vi "运维调试_采配水V4.vi"() -> ()   [LabVIEW 2016, in "PLC.lvlib"]
uses:
  PLC.lvlib
  <vilib>/Plasmionique/MB Master/MB_Master/MB_Master.lvclass
  <vilib>/Utility/miscctls.llb/LVPointTypeDef.ctl
  <vilib>/Plasmionique/MB Master/MB_Master_Serial/MB_Master_Serial.lvclass
  C:/Program Files (x86)/National Instruments/LabVIEW 2016/vi.lib/Plasmionique/MB Master/MB_Master/MB_Master.lvclass
  <vilib>/Instr/_visa.llb/VISA Configure Serial Port (Instr).vi
  <vilib>/NI/Modbus Library/API/Wrapper/Create TCP Slave.vi
  <vilib>/NI/Modbus Library/API/slave/Modbus Slave.lvclass
  <vilib>/Plasmionique/MB Master/MB Master.lvlib
  <vilib>/ptbypt/NI_PtbyPt.lvlib
  <vilib>/NI/Modbus Library/API/Wrapper/API Main.lvlib
panel:
  out "R111":i16 caption="三级水样池润洗时间"
  in  "三级过滤系统":bool
  out "R110":i16 caption="集气时间"
  out "R104":i16 caption="三级润洗时间"
  out "R103":i16 caption="二级润洗时间"
  out "R107":i16 caption="进气时间"
  out "R43":u16
  in  "Y30":bool
  out "Registers":u16[](array[numeric])
  out "R124":i16 caption="加标回收配水时间"
  out "R42":i16
  in  "Y29":bool
  in  "更新程序":bool
  out "R122":i16 caption="二级自来水清洗时间"
  out "R121":i16 caption="一级自来水清洗时间"
  out "R120":i16 caption="过滤自来水清洗时间"
  out "清洗次数":u16
  out "当前启动泵号":u16(ring) items=["1号泵", "2号泵"]
  out "R116":i16 caption="储水时间"
  in  "R113":u16(ring) caption="水箱储水水体" items=["自来水", "水样"]
  out "R112":i16 caption="二级水样池进样超时"
  out "R31":u16
  out "R30":u16
  out "R29":u16
  out "R28":u16
  out "R27":u16
  out "R26":u16
  out "R25":u16
  out "R24":u16
  out "R23":u16
  out "R22":u16
  out "R21":u16
  out "R20":u16
  out "R19":u16
  out "R18":u16
  out "R17":u16
  out "R16":u16
  out "R15":u16
  out "R14":u16
  out "R13":u16
  out "压力传感器":dbl format="%#.2f"
  in  "Y18":bool
  in  "Y17":bool
  in  "Y14":bool
  in  "Y13":bool
  in  "Y1":bool
  in  "Y0":bool
  in  "Y12":bool
  in  "Y11":bool
  in  "Y10":bool
  in  "Y9":bool
  in  "Y8":bool
  in  "Y7":bool
  out "X2":bool caption="X1"
  out "采配水版本号":string
  out "R117":i16 caption="清洗频次设定"
  out "通讯故障":bool
  in  "R100":u16(ring) caption="采水泵工作模式" items=["泵1单泵单管路", "泵2单泵单管路", "潜水泵双泵双管路", "自吸泵双泵双管路"]
  out "X10":bool caption="氨氮水样池液位开关SL3"
  out "X9":bool caption="泵2过载报警_KM2"
  out "X8":bool caption="泵1过载报警_KM1"
  out "X7":bool caption="断电检测_PA"
  out "X6":bool caption="门禁开关_AS"
  out "X5":bool caption="烟雾检测_SA"
  out "X4":bool caption="浸水检测_WIA"
  out "X3":bool caption="水流开关_FS"
  out "X1":bool
  out "X0":bool caption="采样池液位开关_SL1"
  out "R109":i16 caption="外部反冲洗时间"
  out "集成报警信息":string
  out "R108":i16 caption="进样超时时间"
  out "R106":i16 caption="排液时间"
  out "R105":i16 caption="常规模式配水时间"
  out "R102":i16 caption="沉淀时间"
  out "R101":i16 caption="一级润洗时间"
  out "R2":i16
  out "R1":i16
  out "多列列表框":i32(listbox)
  in  "Y6":bool
  in  "Y5":bool
  in  "Y4":bool
  in  "Y3":bool
  in  "Y2":bool
  in  "Y16":bool
  in  "Y15":bool
  in  "返回":bool
  in  "参数设置":bool
  in  "单步启动":bool
  in  "启动":bool
  in  "停止":bool
  # "流程计时："
  # "s"
  # "压力传感器："
  # "MPa"
  # "二级液位开关低_SL2L"
  # "二级液位开关高_SL2H"
  # "S"
  # "S"
  # "S"
  # "S"
  # "S"
  # "S"
  # "S"
  # "S"
  # "S"
  # "S"
  # "S"
  # "次"
  # "S"
  # "S"
  # "S"
  # "S"
  # "S"
  # "S"
  # "单步计时："
  # "s"
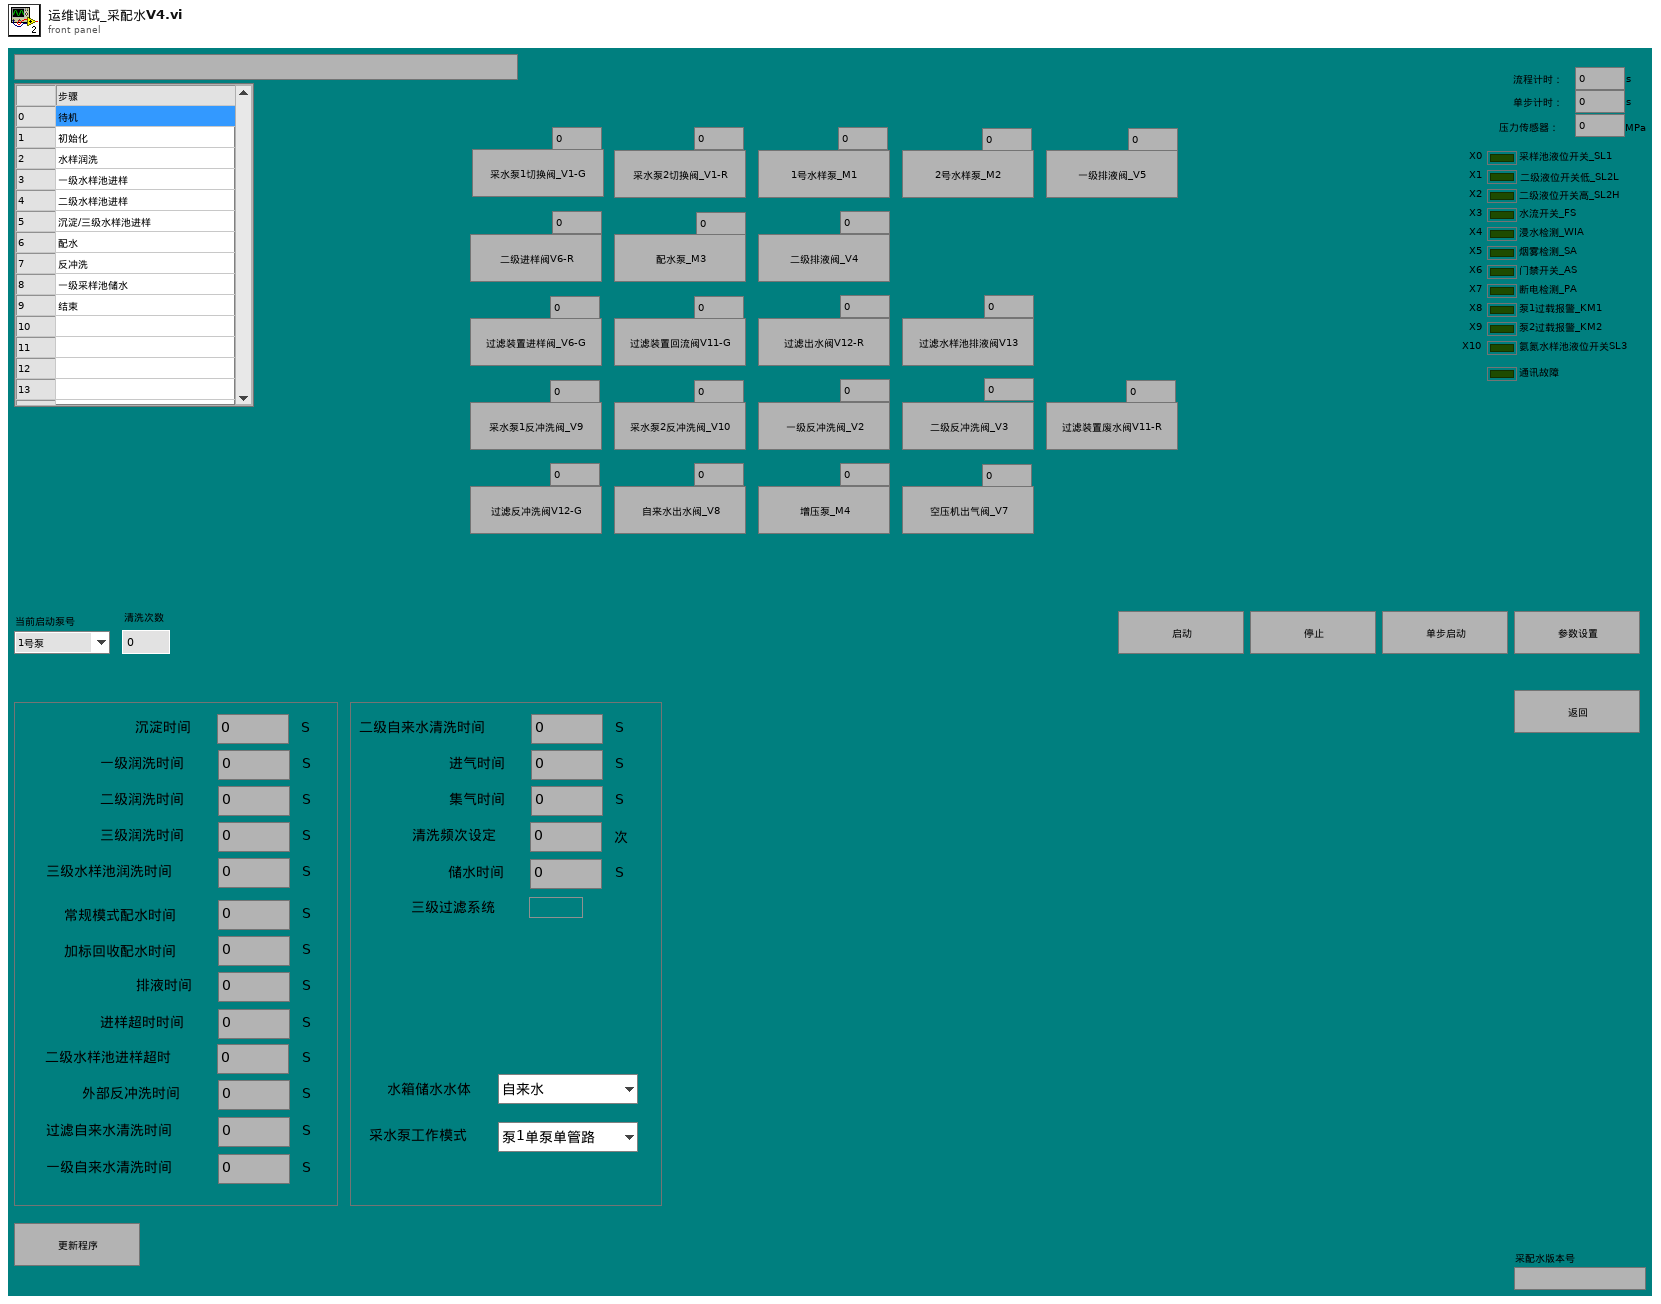
[diagram p1: front panel]
types:
  T1 = typedef "LVPointTypeDef.ctl" = cluster{"Horizontal":i16, "Vertical":i16}
  T2 = cluster{"命令":string, "数据":cluster{"starting address":u16, "holding register value":u16}}
  T3 = cluster{"时间标识":timestamp, "设备":string, "日志信息":string}
  T4 = cluster{"R0":i16, "R1":i16, "R2":i16, "R3":i16, "R4":i16, "R5":i16, "R6":i16, "R7":i16, "R8":i16, "R9":i16, "R10":i16, "R11":i16, "R12":i16, "R13":i16, "R14":i16, "R15":i16, "R16":i16, "R17":i16, "R18":i16, "R19":i16, "R20":i16, "R21":i16, "R22":i16, "R23":i16, "R24":i16, "R25":i16, "R26":i16, "R27":i16, "R28":i16, "R29":i16, "R30":i16, "R31":i16, "R32":i16, "R33":i16, "R34":i16, "R35":i16, "R36":i16, "R37":i16, "R38":i16, "R39":i16, "R40":i16, "R41":i16, "R42":i16, "R43":i16, "R44":i16, "R45":i16, "R46":i16, "R47":i16, "R48":i16, "R49":i16, "R50":i16, "R51":i16, "R52":i16, "R53":i16, "R54":i16, "R55":i16, "R56":i16}
  T5 = cluster{"seconds since 1Jan1904":timestamp, "table输入":string, string, "table输入":string}
  T6 = cluster{"时间标识":timestamp, "设备":string, "日志信息":string, "流程参数":string}
  T7 = cluster{"命令":string, cluster{"starting address":u16, "holding register value":u16}}
  T8 = cluster{"命令":string, "数据":cluster{"starting address":u16, "holding register values":u16[]}}
  T9 = cluster{"命令":string, "data":cluster{"starting address":u16, "coil values":bool[]}}
  T10 = cluster{"测试模式":enum16{"正常测试", "集成干预"}, "参数启用":cluster{"氨氮":bool, "总磷总氮":bool, "CODMn":bool, "CODcr":bool, "多参数":bool, "超标留样":bool, "总氮":bool}}
  T11 = enum32{"Bad", "Idle", "Run top level", "Running"}
  T12 = cluster{"baud rate (bps)":u32, "stop bits":u16, "parity":u16, "flow control":u16, "timeout":u32, "retries":i32}
  T13 = cluster{"starting address":u16, "holding register values":u16[]}
  T14 = cluster{"starting address":u16, "holding register value":u16}
  T15 = cluster{"starting address":u16, "coil values":bool[]}
  T16 = cluster{"Registers[0]":u16, "Registers[1]":u16, "Registers[2]":u16, "Registers[3]":u16, "Registers[4]":u16, "Registers[5]":u16, "Registers[6]":u16, "Registers[7]":u16, "Registers[8]":u16, "Registers[9]":u16, "Registers[10]":u16, "Registers[11]":u16, "Registers[12]":u16, "Registers[13]":u16, "Registers[14]":u16, "Registers[15]":u16, "Registers[16]":u16, "Registers[17]":u16, "Registers[18]":u16, "Registers[19]":u16, "Registers[20]":u16, "Registers[21]":u16, "Registers[22]":u16, "Registers[23]":u16, "Registers[24]":u16, "Registers[25]":u16, "Registers[26]":u16, "Registers[27]":u16, "Registers[28]":u16, "Registers[29]":u16, "Registers[30]":u16, "Registers[31]":u16, "Registers[32]":u16, "Registers[33]":u16, "Registers[34]":u16, "Registers[35]":u16, "Registers[36]":u16, "Registers[37]":u16, "Registers[38]":u16, "Registers[39]":u16, "Registers[40]":u16, "Registers[41]":u16, "Registers[42]":u16, "Registers[43]":u16, "Registers[44]":u16, "Registers[45]":u16, "Registers[46]":u16, "Registers[47]":u16, "Registers[48]":u16, "Registers[49]":u16, "Registers[50]":u16, "Registers[51]":u16, "Registers[52]":u16, "Registers[53]":u16, "Registers[54]":u16, "Registers[55]":u16, "Registers[56]":u16}
  T17 = cluster{"Registers[0]":u16, "Registers[1]":u16, "Registers[2]":u16, "Registers[3]":u16, "Registers[4]":u16, "Registers[5]":u16}
  T18 = cluster{"Registers[0]":u16, "Registers[1]":u16, "Registers[2]":u16, "Registers[3]":u16, "Registers[4]":u16, "Registers[5]":u16, "Registers[6]":u16, "Registers[7]":u16, "Registers[8]":u16, "Registers[9]":u16, "Registers[10]":u16, "Registers[11]":u16, "Registers[12]":u16, "Registers[13]":u16, "Registers[14]":u16, "Registers[15]":u16, "Registers[16]":u16, "Registers[17]":u16, "Registers[18]":u16, "Registers[19]":u16, "Registers[20]":u16, "Registers[21]":u16, "Registers[22]":u16, "Registers[23]":u16, "Registers[24]":u16}
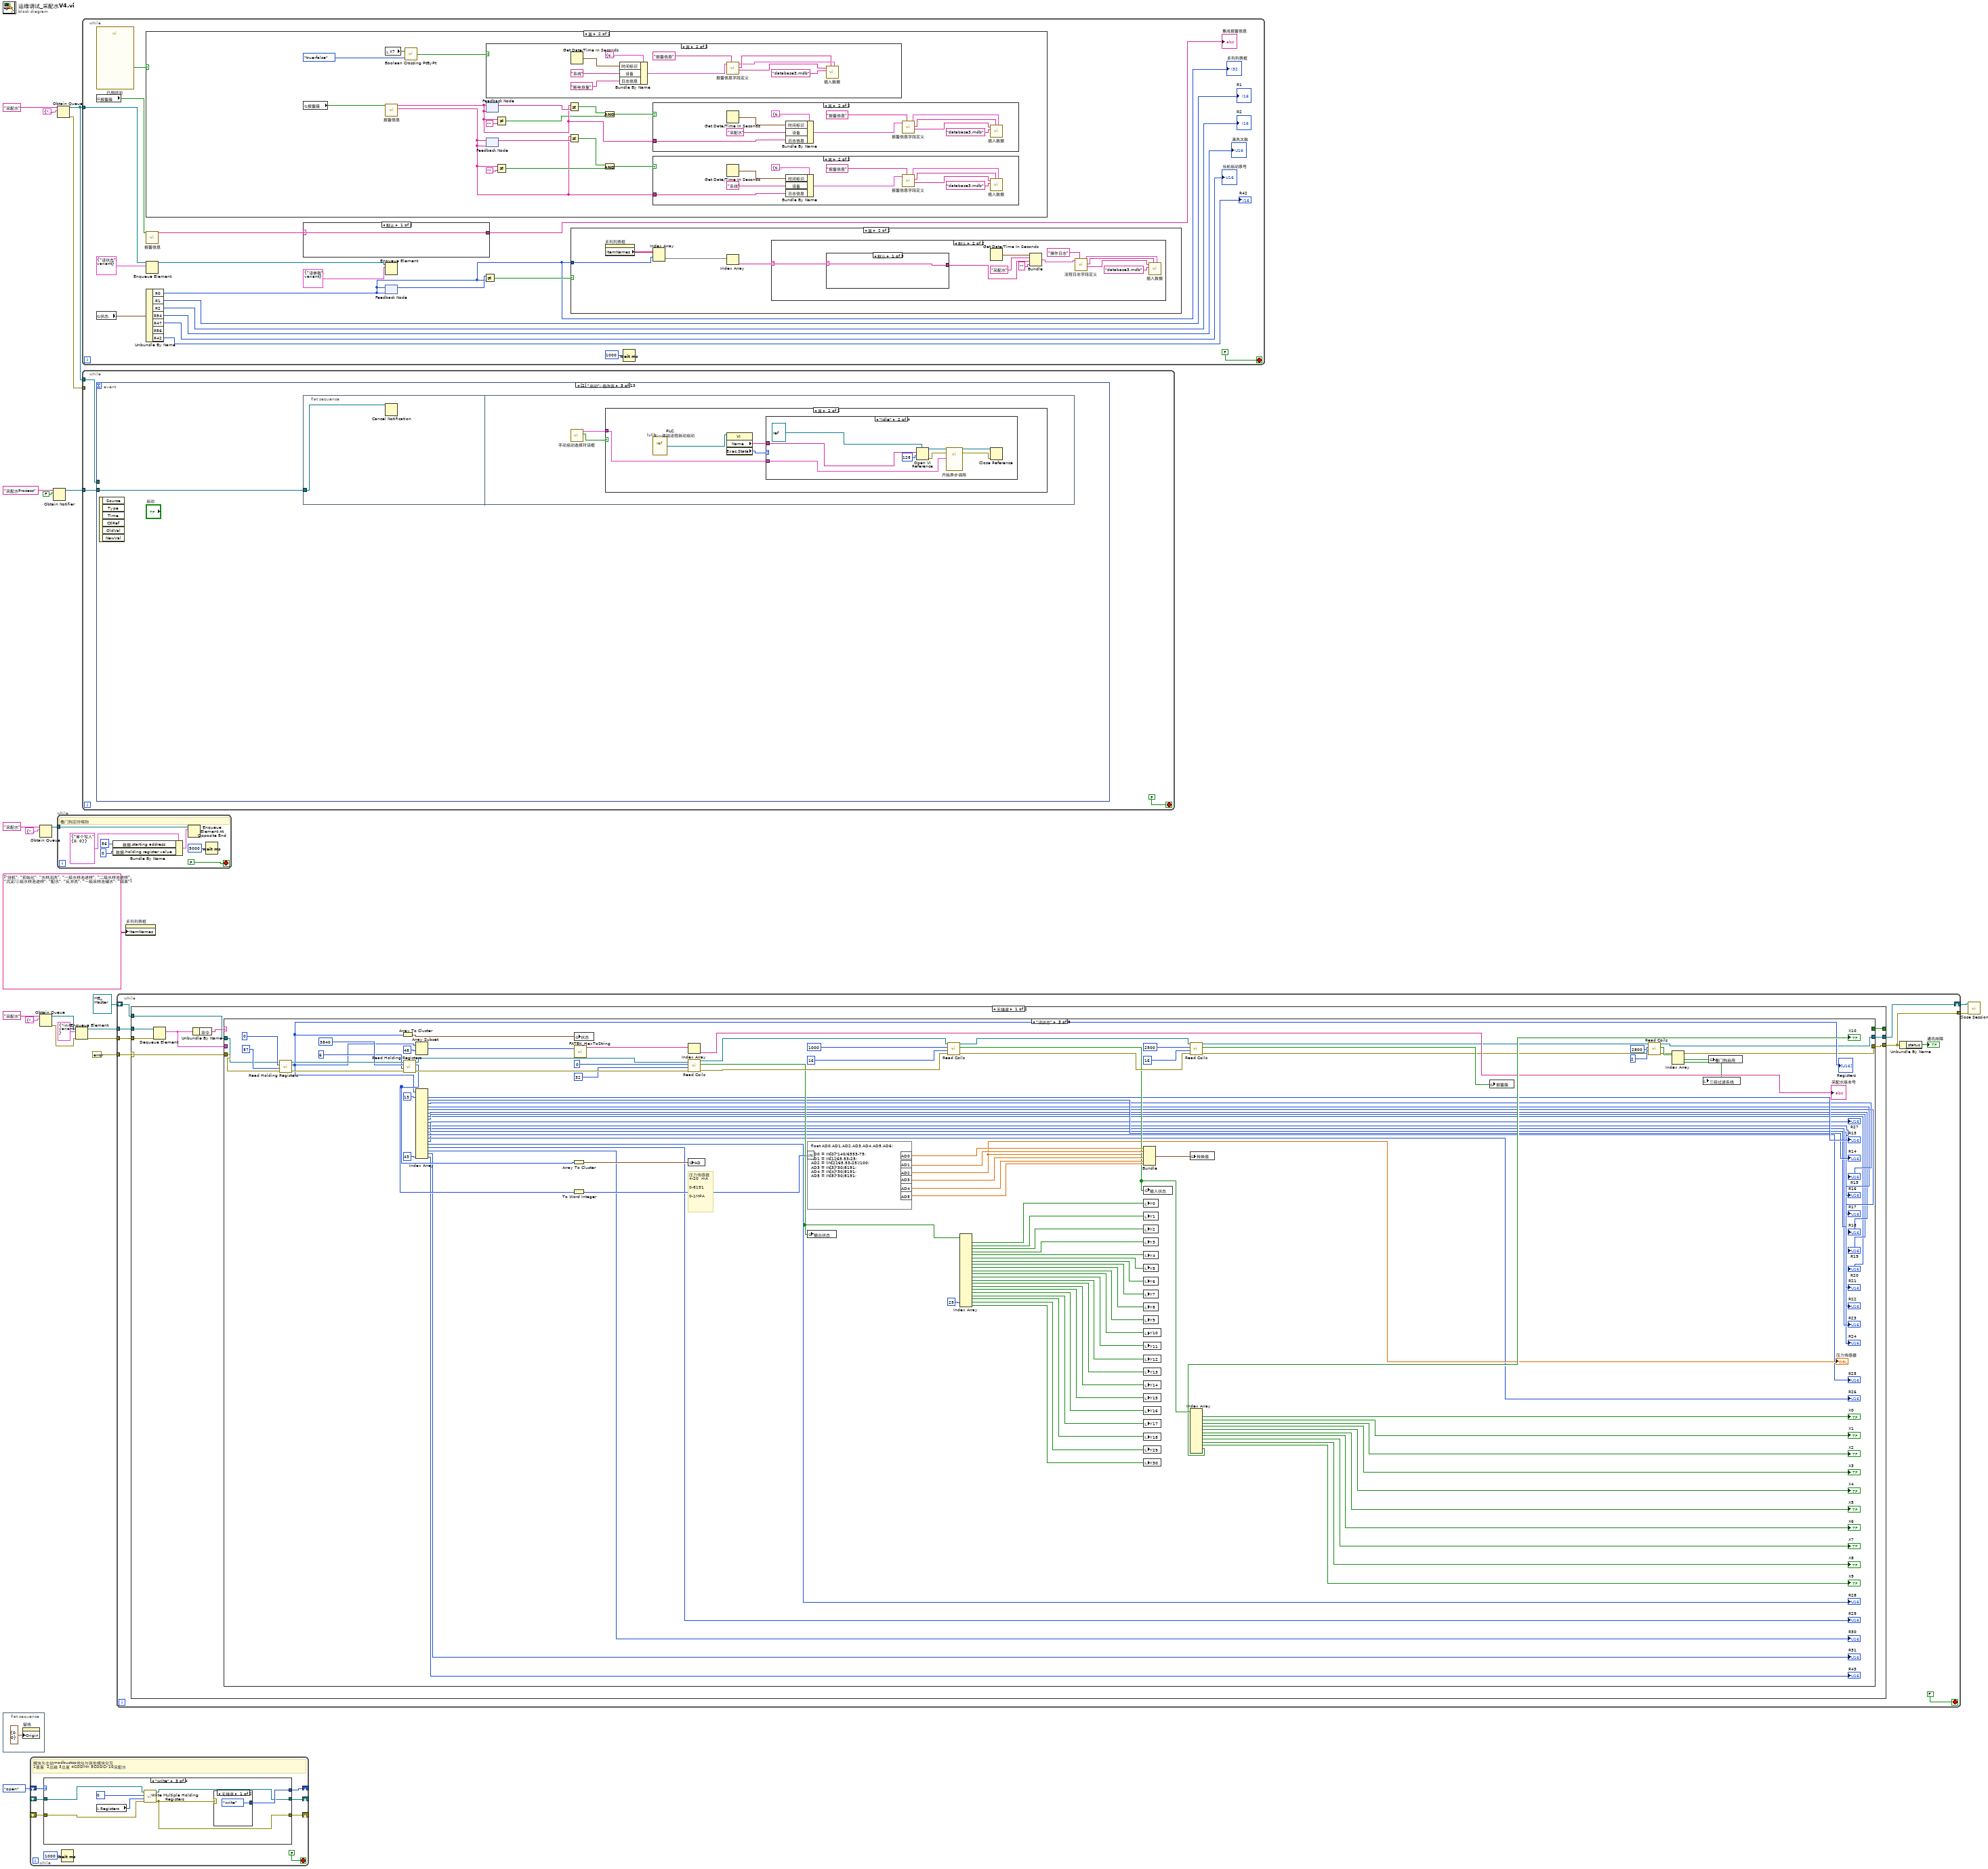
[diagram p0: block diagram]
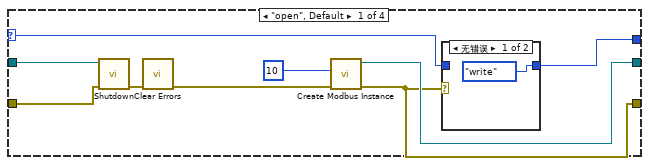
[diagram p2: hidden frame]
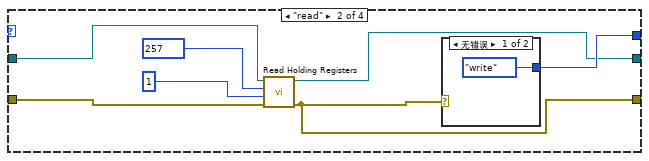
[diagram p4: hidden frame]
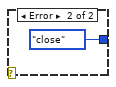
[diagram p5: hidden frame]
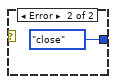
[diagram p6: hidden frame]
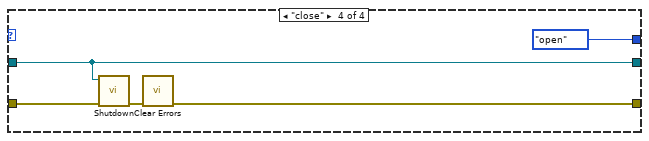
[diagram p7: hidden frame]
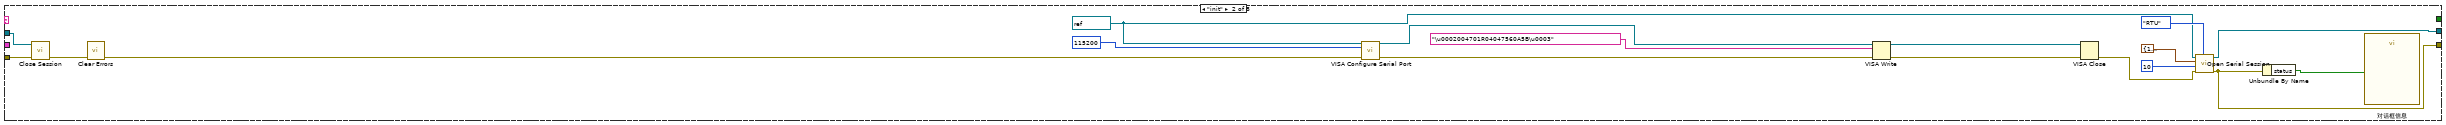
[diagram p9: hidden frame]
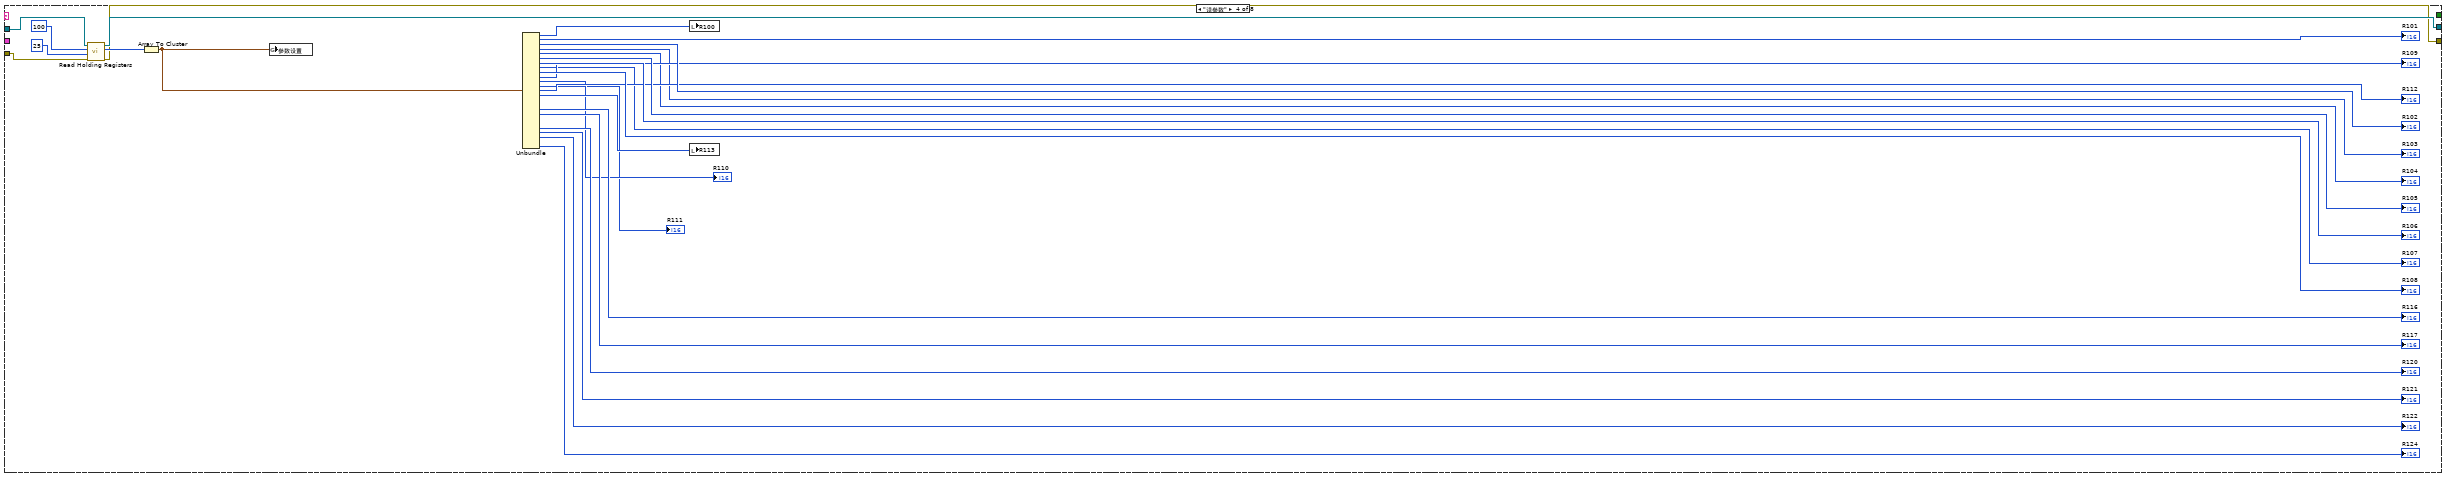
[diagram p10: hidden frame]
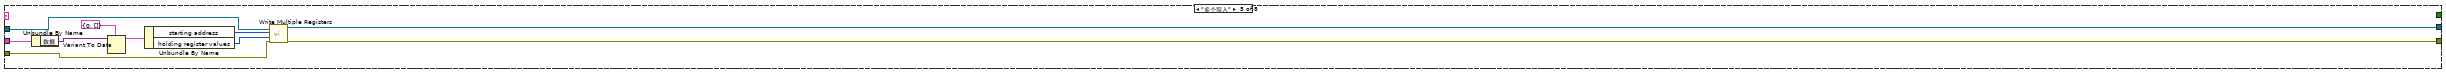
[diagram p11: hidden frame]
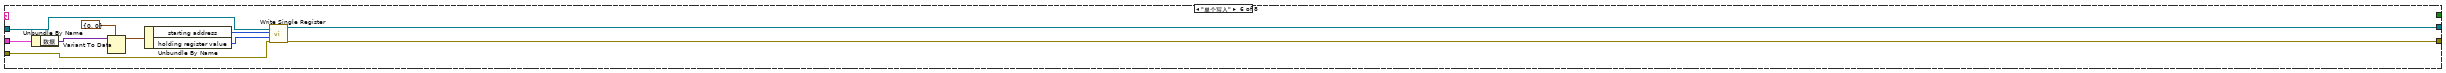
[diagram p12: hidden frame]
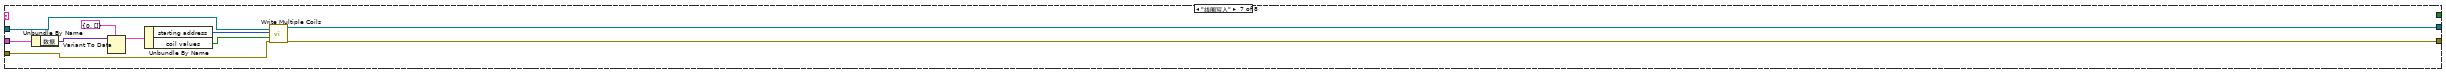
[diagram p13: hidden frame]
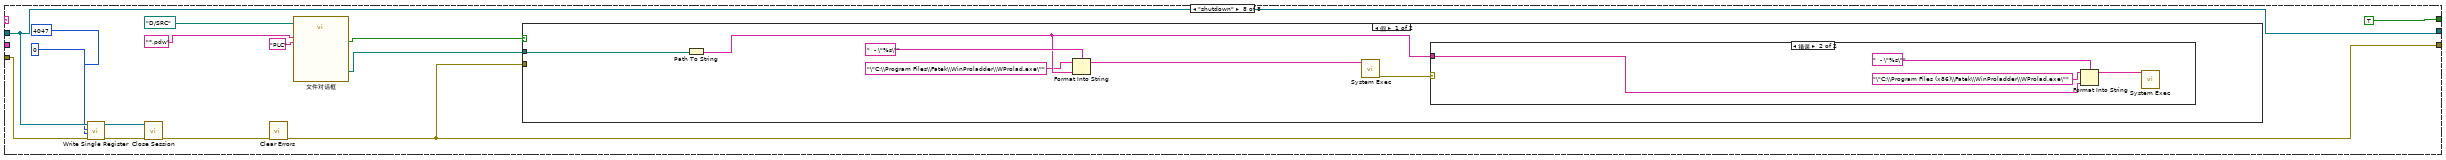
[diagram p14: hidden frame]
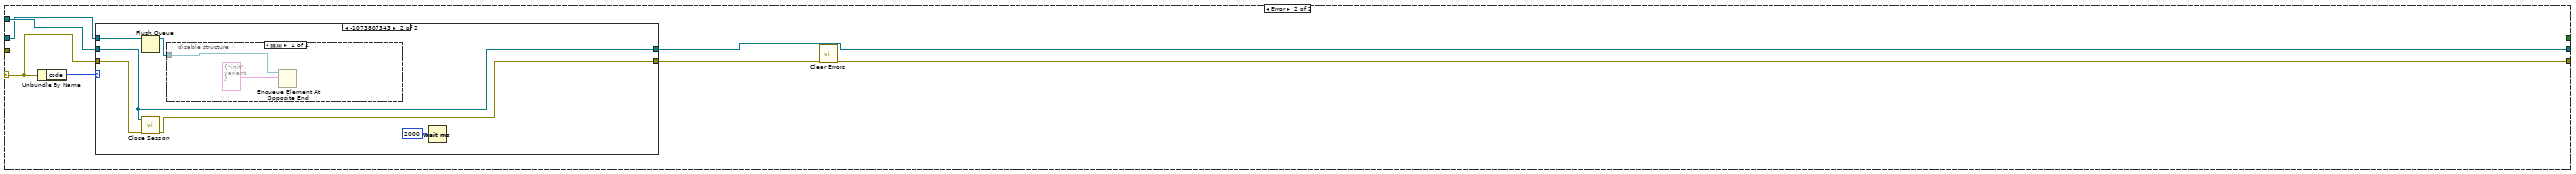
[diagram p17: hidden frame]
diagram:
  n1 = flat-sequence {
    frame #0 {
      n2 = property on="窗格" class="Pane"("Origin"=T1 {"Horizontal"=0, "Vertical"=0} ("原点")) -> ()  [unwired: 2 in, 2 out]
    }
  }
  n3 = while {
    shift-right: [w30] -> _
    shift-left: _ -> [w32]
    shift-right: [w29] -> _
    shift-left: _ -> [w31]
    shift-right: [w26] -> _
    shift-left: enum16{"open", "read", "write", "close"}."open" -> [w27]
    stop <- FALSE stop-if-true
    # "模块为主站modbustcp地址与其他模块交互\n1氨氮  2总磷 3总氮 4CODMn 5CODCr 10采配水"
    n4 = case shown="\"write\"" w27 {
      selector: w27 -> [w41 _ _ _]
      tunnel: w32 -> [w35 w47 w58 w64]
      tunnel: w31 -> [w34 w46 w55 w63]
      tunnel: [w38 w44 w54 w64] -> w30
      tunnel: [w37 w45 w53 w66] -> w29
      tunnel: [w40 w50 w59 enum16{"open", "read", "write", "close"}."open"] -> w26
      frame "open", Default {
        n5 = call-dynamic "Shutdown.vi"("error in"=w34, "Modbus slave in"=w35) -> ("error out"=w33:errorcluster)  [unwired: 9 in]
        n6 = call <vilib>:"Clear Errors.vi"("error in (no error)"=w33) -> ("error out"=w36:errorcluster)  [unwired: 5 in, 1 out]
        n7 = call-poly <vilib>:"Create Modbus Instance.vi"("error in"=w36, "port (502)"=u16 10) -> ("error out"=w37:errorcluster, "TCP slave instance"=w38:refnum<class "Modbus Slave.lvclass">)  [unwired: 8 in]
        n8 = case shown="无错误" w37 {
          tunnel: w41 -> [_ w43]
          tunnel: [enum16{"open", "read", "write", "close"}."write" w43] -> w40
          frame No Error {
          }
          frame Error {
          }
        }
      }
      frame "read" {
        n9 = call-dynamic <vilib>:"Read Holding Registers.vi"("error in"=w46, "number of inputs"=u16 1, "starting address"=u16 257, "Modbus slave in"=w47) -> ("error out"=w45:errorcluster, "Modbus slave out"=w44:refnum<class "Modbus Slave.lvclass">)  [unwired: 5 in, 1 out]
        n10 = case shown="无错误" w45 {
          tunnel: [enum16{"open", "read", "write", "close"}."write" enum16{"open", "read", "write", "close"}."close"] -> w50
          frame No Error {
          }
          frame Error {
          }
        }
      }
      frame "write" {
        n11 = local read "Registers"() -> (w56:u16[])
        n12 = call-dynamic "Write Multiple Holding Registers.vi"("error in"=w55, "registers to write"=w56, "starting address"=u16 0, "Modbus slave in"=w58) -> ("error out"=w53:errorcluster, "Modbus slave out"=w54:refnum<class "Modbus Slave.lvclass">)  [unwired: 6 in]
        n13 = case shown="无错误" w53 {
          tunnel: [enum16{"open", "read", "write", "close"}."write" enum16{"open", "read", "write", "close"}."close"] -> w59
          frame No Error {
          }
          frame Error {
          }
        }
      }
      frame "close" {
        n14 = call-dynamic "Shutdown.vi"("error in"=w63, "Modbus slave in"=w64) -> ("error out"=w62:errorcluster)  [unwired: 9 in]
        n15 = call <vilib>:"Clear Errors.vi"("error in (no error)"=w62) -> ("error out"=w66:errorcluster)  [unwired: 5 in, 1 out]
      }
    }
    n16 = Wait (ms)(milliseconds to wait=u32 1000 ("等待时间（毫秒）")) -> ()  [unwired: 1 out]
  }
  n17 = Obtain Queue(name (unnamed)="采配水" ("名称（未命名）"), element data type=cluster{"命令":string, "数据":variant} {"命令"="", "数据"=variant}) -> (queue out=w2:refnum<queue>)  [unwired: 3 in, 2 out]
  n18 = Obtain Queue(name (unnamed)="采配水" ("名称（未命名）"), element data type=cluster{"命令":string, "数据":variant} {"命令"="", "数据"=variant}) -> (queue out=w13:refnum<queue>, error out=w12:errorcluster)  [unwired: 3 in, 1 out]
  n19 = Obtain Notifier(name (unnamed)="采配水Process" ("名称（未命名）"), notification data type=FALSE) -> (notifier out=w16:refnum<notifier>)  [unwired: 2 in, 2 out]
  n20 = while {
    tunnel: w2 -> [w71]
    stop <- FALSE stop-if-true
    # "看门狗定时喂狗"
    n21 = Bundle By Name(cluster=T2 {"命令"="单个写入", "数据"={"starting address"=0, "holding register value"=0}} ("元素"), "数据.starting address"=u16 56, "数据.holding register value"=u16 0) -> (w72:T2)
    n22 = Enqueue Element At Opposite End(queue=w71, element=w72) -> ()  [unwired: 2 in, 3 out]
    n23 = Wait (ms)(milliseconds to wait=u32 5000 ("等待时间（毫秒）")) -> ()  [unwired: 1 out]
  }
  n24 = Obtain Queue(name (unnamed)="采配水" ("名称（未命名）"), element data type=cluster{"命令":string, "数据":variant} {"命令"="", "数据"=variant}) -> (queue out=w20:refnum<queue>, error out=w21:errorcluster)  [unwired: 3 in, 1 out]
  n25 = Enqueue Element(queue=w13, element=cluster{"命令":string, "数据":variant} {"命令"="init", "数据"=variant} ("元素"), error in (no error)=w12) -> (queue out=w8:refnum<queue>, error out=w10:errorcluster)  [unwired: 1 in, 1 out]
  n26 = while {
    tunnel: w20 -> [w91]
    stop <- FALSE stop-if-true
    n27 = call "已用时间"() -> ("Time has Elapsed"=w83:bool)  [unwired: 12 in, 7 out]
    n28 = global read "采配水全局变量.vi" "报警簇"() -> (w85:bool[])
    n29 = global read "采配水全局变量.vi" "状态"() -> (w89:T4)
    n30 = case shown="真" w83 {
      frame False {
      }
      frame True {
        n31 = global read "采配水全局变量.vi" "报警簇"() -> (w108:bool[])
        n32 = local read "X7"() -> (w95:bool)
        n33 = call "报警信息.vi"("报警簇"=w108) -> ("系统报警信息"=w97:string, "采配水报警信息"=w104:string)  [unwired: 9 in]
        n34 = call <vilib>:"Boolean Crossing PtByPt.vi"("direction"=enum16{"either", "false-true", "true-false"}."true-false", "input"=w95) -> ("crossing"=w93:bool)  [unwired: 1 in]
        n35 = case shown="真" w93 {
          frame False {
          }
          frame True {
            n36 = Get Date/Time In Seconds() -> (seconds since 1Jan1904=w117:timestamp)
            n37 = Bundle By Name(cluster=T3 {"时间标识"=timestamp(0 s since 1904-01-01), "设备"="", "日志信息"=""} ("data in"), "时间标识"=w117, "设备"="系统", "日志信息"="断电恢复") -> (w116:T3)
            n38 = call "报警信息字段定义.vi"("table输入"="报警信息", "data in"=w116) -> ("table输出"=w112:string, "columns"=w111:string[], "data out"=w110:T3)  [unwired: 7 in]
            n39 = call "插入数据.vi"("data"=w110, "columns"=w111, "database"="database3.mdb", "table"=w112) -> ()  [unwired: 7 in, 1 out]
          }
        }
        n40 = feedback #1(w104) -> (w107:string)
        n41 = feedback-in #1(w104) -> ()
        n42 = feedback #2(w97) -> (w98:string)
        n43 = feedback-in #2(w97) -> ()
        n44 = Not Equal?(x=w104, y="") -> (x != y?=w102:bool)
        n45 = Not Equal?(x=w97, y="") -> (x != y?=w101:bool)
        n46 = Not Equal?(x=w104, y=w107) -> (x != y?=w106:bool)
        n47 = Not Equal?(x=w97, y=w98) -> (x != y?=w99:bool)
        n48 = And(x=w106, y=w102) -> (x .and. y?=w105:bool)
        n49 = And(x=w99, y=w101) -> (x .and. y?=w96:bool)
        n50 = case shown="真" w105 {
          tunnel: w104 -> [_ w129]
          frame False {
          }
          frame True {
            n51 = Get Date/Time In Seconds() -> (seconds since 1Jan1904=w131:timestamp)
            n52 = Bundle By Name(cluster=T3 {"时间标识"=timestamp(0 s since 1904-01-01), "设备"="", "日志信息"=""} ("data in"), "时间标识"=w131, "设备"="采配水", "日志信息"=w129) -> (w132:T3)
            n53 = call "报警信息字段定义.vi"("table输入"="报警信息", "data in"=w132) -> ("table输出"=w136:string, "columns"=w137:string[], "data out"=w138:T3)  [unwired: 7 in]
            n54 = call "插入数据.vi"("data"=w138, "columns"=w137, "database"="database3.mdb", "table"=w136) -> ()  [unwired: 7 in, 1 out]
          }
        }
        n55 = case shown="真" w96 {
          tunnel: w97 -> [_ w119]
          frame False {
          }
          frame True {
            n56 = Get Date/Time In Seconds() -> (seconds since 1Jan1904=w121:timestamp)
            n57 = Bundle By Name(cluster=T3 {"时间标识"=timestamp(0 s since 1904-01-01), "设备"="", "日志信息"=""} ("data in"), "时间标识"=w121, "设备"="系统", "日志信息"=w119) -> (w122:T3)
            n58 = call "报警信息字段定义.vi"("table输入"="报警信息", "data in"=w122) -> ("table输出"=w126:string, "columns"=w127:string[], "data out"=w128:T3)  [unwired: 7 in]
            n59 = call "插入数据.vi"("data"=w128, "columns"=w127, "database"="database3.mdb", "table"=w126) -> ()  [unwired: 7 in, 1 out]
          }
        }
      }
    }
    n60 = call "报警信息.vi"("报警簇"=w85) -> ("采配水报警信息"=w77:string)  [unwired: 9 in, 1 out]
    n61 = Enqueue Element(queue=w91, element=cluster{"命令":string, "数据":variant} {"命令"="读状态", "数据"=variant} ("元素")) -> (queue out=w80:refnum<queue>)  [unwired: 2 in, 2 out]
    n62 = Unbundle By Name(w89) -> ("R0"=w78:i16, "R1"=→"R1":i16, "R2"=→"R2":i16, "R54"=→"清洗次数":i16, "R47"=→"当前启动泵号":i16, "R42"=→"R42":i16)  [unwired: 1 out]
    "多列列表框" <- w78
    n63 = case shown="默认" w77 {
      selector: w77 -> [w139 _]
      tunnel: [w139 w140] -> w84
      frame Default {
      }
      frame "" {
        n64 = global read "采配水全局变量.vi" "运行状态显示"() -> (w140:string)
      }
    }
    "集成报警信息" <- w84
    n65 = Enqueue Element(queue=w80, element=cluster{"命令":string, "数据":variant} {"命令"="读参数", "数据"=variant} ("元素")) -> ()  [unwired: 2 in, 3 out]
    n66 = feedback-in #3(w78) -> ()
    n67 = feedback #3(w78) -> (w79:i16)
    n68 = Not Equal?(x=w79, y=w78) -> (x != y?=w86:bool)
    n69 = case shown="真" w86 {
      tunnel: w78 -> [_ w143]
      frame False {
      }
      frame True {
        n70 = property on="多列列表框" class="MCListbox (严格)"() -> ("ItemNames"=w144:string[][])  [unwired: 2 in, 2 out]
        n71 = Index Array(array=w144, index (row)=w143) -> (element=w142:string[])  [unwired: 1 in]
        n72 = Index Array(array=w142) -> (element=w141:string)  [unwired: 1 in]
        n73 = case shown="默认" w141 {
          selector: w141 -> [_ w146]
          frame "待机" {
          }
          frame Default {
            n74 = case shown="默认" w146 {
              selector: w146 -> [w156 _ _]
              tunnel: [w156 "-->>启动" "-->>结束"] -> w145
              frame Default {
              }
              frame "初始化" {
              }
              frame "结束" {
              }
            }
            n75 = Get Date/Time In Seconds() -> (seconds since 1Jan1904=w150:timestamp)
            n76 = Bundle("seconds since 1Jan1904"=w150, "table输入"="采配水", w145, "table输入"="") -> (w148:T5)  [unwired: 1 in]
            n77 = call "流程日志字段定义.vi"("table输入"="操作日志", "data in"=w148) -> ("table输出"=w153:string, "columns"=w154:string[], "data out"=w155:T6)  [unwired: 7 in]
            n78 = call "插入数据.vi"("data"=w155, "columns"=w154, "database"="database3.mdb", "table"=w153) -> ()  [unwired: 7 in, 1 out]
          }
        }
      }
    }
    n79 = Wait (ms)(milliseconds to wait=u32 1000 ("等待时间（毫秒）")) -> ()  [unwired: 1 out]
  }
  n80 = while {
    tunnel: w20 -> [w160]
    tunnel: w21 -> [_]
    tunnel: w16 -> [w159]
    stop <- FALSE stop-if-true
    n81 = event shown="[2] \"启动\": 值改变" {
      selector: _ -> [_ _ _ _ _ _ _ _ _ _ _ _ _]
      dyn-events: _ -> [_ _ _ _ _ _ _ _ _ _ _ _ _]
      timeout: _ -> [_ _ _ _ _ _ _ _ _ _ _ _ _]
      tunnel: w160 -> [_ w164 _ w186 w205 w214 w219 _ _ _ w254 w257 w263]
      tunnel: w159 -> [_ w163 w166 _ _ _ _ _ _ _ _ _ _]
      event Timeout {
        n82 = event-data() -> ()  [unwired: 1 in, 3 out]
      }
      event "停止": Value Change {
        n83 = event-data() -> ()  [unwired: 1 in, 6 out]
        n84 = Send Notification(notification=TRUE ("通知"), notifier=w163) -> ()  [unwired: 1 in, 2 out]
        n85 = Enqueue Element At Opposite End(queue=w164, element=T7 {"命令"="单个写入", {"starting address"=300, "holding register value"=2}} ("元素")) -> ()  [unwired: 2 in, 3 out]
      }
      event "启动": Value Change {
        n86 = event-data() -> ()  [unwired: 1 in, 6 out]
        n87 = flat-sequence {
          tunnel: w166 -> [w167]
          frame #0 {
            n88 = Cancel Notification(0:w167) -> ()  [unwired: 1 in, 3 out]
          }
          frame #1 {
            n89 = call "手动启动选择对话框.vi"() -> ("确定"=w169:bool, "输出簇"=w168:T10)  [unwired: 10 in]
            n90 = case shown="真" w169 {
              tunnel: w168 -> [_ w170]
              frame False {
              }
              frame True {
                n91 = vi-ref "PLC.lvlib:一体站流程自动启动.vi"() -> (w173:refnum<vi>)
                n92 = property class="VI"(reference=w173) -> ("Name"=w172:string, "Exec.State"=w171:T11)  [unwired: 1 in, 2 out]
                n93 = case shown="\"Idle\"" w171 {
                  tunnel: w172 -> [_ w181 _ _]
                  tunnel: w170 -> [_ w175 _ _]
                  frame "Bad", Default {
                  }
                  frame "Idle" {
                    n94 = Open VI Reference(type specifier VI Refnum (for type only)=refnum<vi> refnum, vi path=w181, options=128 ("选项")) -> (vi reference=w179:refnum<vi>, error out=w177:errorcluster)  [unwired: 3 in]
                    n95 = call-by-ref "开始异步调用"(reference=w179, error in=w177, "参数"=w175) -> (reference out=w178:refnum<vi>, error out=w176:errorcluster)  [unwired: 11 in]
                    n96 = Close Reference(reference=w178, error in (no error)=w176) -> ()  [unwired: 1 out]
                  }
                  frame "Run top level" {
                  }
                  frame "Running" {
                    n97 = One Button Dialog(message="流程已启动，无需重复启动！" ("消息")) -> ()  [unwired: 1 in, 1 out]
                  }
                }
              }
            }
          }
        }
      }
      event "单步启动": Value Change {
        n98 = event-data() -> ()  [unwired: 1 in, 6 out]
        n99 = call "单步启动对话框.vi"() -> ("单步启动步骤输出"=w183:u16)  [unwired: 11 in]
        n100 = Bundle By Name(cluster=T2 {"命令"="单个写入", "数据"={"starting address"=301, "holding register value"=0}} ("元素"), "数据.holding register value"=w183) -> (w184:T2)
        n101 = Enqueue Element At Opposite End(queue=w186, element=w184) -> ()  [unwired: 2 in, 3 out]
      }
      event "R101", "R102", "R105", "R106", "R108", "R109", "R100", "R112", "R113", "R103", "R104", "R107", "R110", "R111": Value Change {
        n102 = event-data() -> ()  [unwired: 1 in, 6 out]
        n103 = local read "R111"() -> (w187:i16)
        n104 = local read "R110"() -> (w188:i16)
        n105 = local read "R101"() -> (w201:i16)
        n106 = local read "R102"() -> (w200:i16)
        n107 = local read "R103"() -> (w190:i16)
        n108 = local read "R104"() -> (w189:i16)
        n109 = local read "R105"() -> (w199:i16)
        n110 = local read "R106"() -> (w198:i16)
        n111 = local read "R107"() -> (w197:i16)
        n112 = local read "R108"() -> (w196:i16)
        n113 = local read "R109"() -> (w194:i16)
        n114 = local read "R112"() -> (w192:i16)
        n115 = Build Array("R100", w201, w200, w190, w189, w199, w198, w197, w196, w194, w188, w187, w192, "R113") -> (w193:u16[])
        n116 = Bundle By Name(cluster=T8 {"命令"="多个写入", "数据"={"starting address"=0, "holding register values"=[]}} ("元素"), "数据.starting address"=u16 100, "数据.holding register values"=w193) -> (w202:T8)
        n117 = Enqueue Element At Opposite End(queue=w205, element=w202) -> ()  [unwired: 2 in, 3 out]
      }
      event "R116", "R117", "R120", "R121", "R122": Value Change {
        n118 = event-data() -> ()  [unwired: 1 in, 6 out]
        n119 = local read "R116"() -> (w212:i16)
        n120 = local read "R117"() -> (w211:i16)
        n121 = local read "R120"() -> (w210:i16)
        n122 = local read "R121"() -> (w209:i16)
        n123 = local read "R122"() -> (w208:i16)
        n124 = Build Array(w212, w211, i16 0 ("元素"), i16 0 ("R116"), w210, w209, w208) -> (w213:i16[])
        n125 = Bundle By Name(cluster=T8 {"命令"="多个写入", "数据"={"starting address"=0, "holding register values"=[]}} ("元素"), "数据.starting address"=u16 116, "数据.holding register values"=w213) -> (w215:T8)
        n126 = Enqueue Element At Opposite End(queue=w214, element=w215) -> ()  [unwired: 2 in, 3 out]
      }
      event "R124": Value Change {
        n127 = event-data() -> ("NewVal"=w218:i16)  [unwired: 1 in, 5 out]
        n128 = Build Array(w218) -> (w220:i16[])
        n129 = Bundle By Name(cluster=T8 {"命令"="多个写入", "数据"={"starting address"=0, "holding register values"=[]}} ("元素"), "数据.starting address"=u16 124, "数据.holding register values"=w220) -> (w221:T8)
        n130 = Enqueue Element At Opposite End(queue=w219, element=w221) -> ()  [unwired: 2 in, 3 out]
      }
      event "R101", "R102", "R105", "R106", "R108", "R109", "R117", "R116", "R112", "R120", "R121", "R122", "R124", "R107", "R103", "R104", "R110", "R111": Mouse Down {
        n131 = event-data() -> ("CtlRef"=w227:refnum<vi>)  [unwired: 1 in, 7 out]
        n132 = property class="DigNum (严格)"(reference=w227) -> (reference out=w225:refnum<vi>, "Value"=w226:i16)  [unwired: 1 in, 1 out]
        n133 = call "数字键盘.vi"("OldNumber"=w226) -> ("NewNumber"=w224:sgl)
        n134 = property class="DigNum (严格)"(reference=w225, "Val(Sgnl)"=w224) -> ()  [unwired: 1 in, 2 out]
      }
      event "参数设置": Value Change {
        n135 = event-data() -> ()  [unwired: 1 in, 6 out]
        n136 = property on="窗格" class="Pane"("Origin"=T1 {"Horizontal"=0, "Vertical"=628} ("原点")) -> ()  [unwired: 2 in, 2 out]
      }
      event "返回": Value Change {
        n137 = event-data() -> ()  [unwired: 1 in, 6 out]
        n138 = property on="窗格" class="Pane"("Origin"=T1 {"Horizontal"=0, "Vertical"=0} ("原点")) -> ()  [unwired: 2 in, 2 out]
      }
      event "Y15", "Y16", "Y2", "Y3", "Y4", "Y5", "Y6", "Y7", "Y8", "Y9", "Y10", "Y11", "Y12", "Y0", "Y1", "Y13", "Y14", "Y18", "Y17", "Y29", "Y30": Value Change {
        n139 = event-data() -> ()  [unwired: 1 in, 6 out]
        n140 = Build Array("Y0", "Y1", "Y2", "Y3", "Y4", "Y5", "Y6", "Y7", "Y8", "Y9", "Y10", "Y11", "Y12", "Y13", "Y14", "Y15", "Y16", "Y17", "Y18", "Y29", "Y30") -> (w247:bool[])
        n141 = Bundle By Name(cluster=T9 {"命令"="线圈写入", "data"={"starting address"=2400, "coil values"=[]}} ("元素"), "data.coil values"=w247) -> (w248:T9)
        n142 = Enqueue Element(queue=w254, element=w248) -> ()  [unwired: 2 in, 3 out]
      }
      event "三级过滤系统": Value Change {
        n143 = event-data() -> ()  [unwired: 1 in, 6 out]
        n144 = Build Array("三级过滤系统") -> (w255:bool[])
        n145 = Bundle By Name(cluster=T9 {"命令"="线圈写入", "data"={"starting address"=2801, "coil values"=[]}} ("元素"), "data.coil values"=w255) -> (w258:T9)
        n146 = Enqueue Element(queue=w257, element=w258) -> ()  [unwired: 2 in, 3 out]
      }
      event "更新程序": Value Change {
        n147 = event-data() -> ("NewVal"=w260:bool)  [unwired: 1 in, 5 out]
        n148 = Flush Queue(queue=w263) -> (queue out=w261:refnum<queue>)  [unwired: 1 in, 2 out]
        n149 = case shown="真" w260 {
          tunnel: [cluster{"命令":string, "数据":variant} {"命令"="init", "数据"=variant} ("元素") w267] -> w262
          frame False {
          }
          frame True {
            n150 = Two Button Dialog(message="警告，非专业人士请勿进行此操作！！！\n请确认是否释放串口？" ("消息")) -> (T button?=w266:bool)  [unwired: 2 in]
            n151 = case shown="真" w266 {
              tunnel: [_ cluster{"命令":string, "数据":variant} {"命令"="shutdown", "数据"=variant} ("元素")] -> w267
              frame False {
                n152 = local write "更新程序"(FALSE ("释放串口")) -> ()
              }
              frame True {
              }
            }
          }
        }
        n153 = Enqueue Element(queue=w261, element=w262) -> ()  [unwired: 2 in, 3 out]
      }
    }
  }
  n154 = while {
    tunnel: w8 -> [w274]
    tunnel: w10 -> [w273]
    shift-right: [w277] -> w5
    shift-left: refnum<class "MB_Master.lvclass"> refnum ("MB session in") -> [w276]
    tunnel: errorcluster {"status"=FALSE, "code"=0, "source"=""} ("error out") -> [w275]
    tunnel: [w272] -> w6
    stop <- FALSE stop-if-true
    n155 = case shown="无错误" w275 {
      selector: w275 -> [w283 w496]
      tunnel: [w286 w495] -> w277
      tunnel: w276 -> [w285 w497]
      tunnel: [w284 w493] -> w272
      tunnel: w274 -> [w280 w492]
      tunnel: w273 -> [w279 _]
      tunnel: [w281 _] -> _
      frame No Error {
        n156 = Dequeue Element(queue=w280, error in (no error)=w279) -> (element=w278:cluster{"命令":string, "数据":variant})  [unwired: 1 in, 3 out]
        n157 = Unbundle By Name(w278) -> ("命令"=w282:string)
        n158 = case shown="\"读状态\"" w282 {
          tunnel: [w288 w301 w317 w432 w444 w454 w464 w479] -> w286
          tunnel: w285 -> [w288 w303 w399 w437 w447 w457 w467 w479]
          tunnel: [w287 w302 w307 w431 w445 w455 w465 w470] -> w284
          tunnel: w283 -> [w287 w305 w402 w436 w446 w456 w466 w475]
          tunnel: [_ _ _ _ _ _ _ TRUE] -> w281
          tunnel: w278 -> [_ _ _ _ w443 w453 w463 _]
          frame "idle", Default {
          }
          frame "init" {
            w292 = refnum<visa-resource-name> "COM3" ("VISA resource name")
            n159 = call-dynamic "Close Session.vi"("error in (no error)"=w305, "MB session in"=w303) -> ("error out"=w304:errorcluster)  [unwired: 9 in]
            n160 = call <vilib>:"Clear Errors.vi"("error in (no error)"=w304) -> ("error out"=w290:errorcluster)  [unwired: 5 in, 1 out]
            n161 = call-poly "VISA Configure Serial Port"("VISA resource name"=w292, "baud rate (9600)"=u32 115200, "error in (no error)"=w290) -> ("VISA resource name out"=w297:refnum<visa-resource-name>, "error out"=w296:errorcluster)  [unwired: 11 in]
            n162 = VISA Write(VISA resource name=w297, write buffer="\u0002004701R04047560A5B\u0003" ("写入缓冲区"), error in (no error)=w296) -> (VISA resource name out=w295:refnum<visa-resource-name>, error out=w294:errorcluster)  [unwired: 1 out]
            n163 = VISA Close(VISA resource name=w295, error in (no error)=w294) -> (error out=w289:errorcluster)
            n164 = call <vilib>:"Open Serial Session.vi"("Mode (RTU)"=enum16{"RTU", "ASCII"}."RTU", "Error in"=w289, "Slave ID"=u8 10, "Serial Config"=T12 {"baud rate (bps)"=115200, "stop bits"=10, "parity"=0, "flow control"=0, "timeout"=500, "retries"=1}, "VISA Resource"=w292) -> ("Error out"=w302:errorcluster, "MB_Serial session"=w301:refnum<class "MB_Master_Serial.lvclass">)  [unwired: 5 in]
            n165 = Unbundle By Name(w302) -> ("status"=w306:bool)
            n166 = call "对话框信息"("Enable"=w306) -> ()  [unwired: 9 in, 2 out]
          }
          frame "读状态" {
            # "压力传感器\n4-20  mA \n \n0-8191\n\n0-1MPA"
            n167 = call <vilib>:"Read Holding Registers.vi"("error in (no error)"=w402, "quantity"=u16 57 ("number of holding registers"), "starting address"=u16 0, "MB session in"=w399) -> ("error out"=w397:errorcluster, "Registers"=w342:u16[], "MB session out"=w398:refnum<class "MB_Master.lvclass">)  [unwired: 5 in]
            "Registers" <- w342
            n168 = Array To Cluster(array=w342) -> (cluster=w321:T16)
            n169 = call <vilib>:"Read Holding Registers.vi"("error in (no error)"=w397, "quantity"=u16 6 ("number of holding registers"), "starting address"=u16 3840, "MB session in"=w398) -> ("error out"=w393:errorcluster, "Registers"=w371:u16[], "MB session out"=w394:refnum<class "MB_Master.lvclass">)  [unwired: 5 in]
            n170 = Array Subset(array=w342, index=48 ("索引")) -> (w368:u16[])  [unwired: 1 in]
            n171 = Index Array(array=w342, index #1=13 ("索引"), index #20=43 ("索引")) -> (element #1=→"R13":u16, element #2=→"R14":u16, element #3=→"R15":u16, element #4=→"R16":u16, element #5=→"R17":u16, element #6=→"R18":u16, element #7=→"R19":u16, element #8=→"R20":u16, element #9=→"R21":u16, element #10=→"R22":u16, element #11=→"R23":u16, element #12=→"R24":u16, element #13=→"R25":u16, element #14=→"R26":u16, element #15=→"R27":u16, element #16=→"R28":u16, element #17=→"R29":u16, element #18=→"R30":u16, element #19=→"R31":u16, element #20=→"R43":u16)  [unwired: 18 in]
            n172 = Array To Cluster(array=w371) -> (cluster=w409:T17)
            n173 = To Word Integer(number=w371) -> (16bit integer=w370:i16[])
            n174 = global write "采配水全局变量.vi" "状态"(w321) -> ()
            n175 = call "FATEK_HexToString.vi"("数组"=w368) -> ("STRING"=w367:string[])  [unwired: 10 in]
            n176 = Index Array(array=w367) -> (element=→"采配水版本号":string)  [unwired: 1 in]
            n177 = call <vilib>:"Read Coils.vi"("error in (no error)"=w393, "quantity"=u16 32 ("number of coils"), "starting address"=u16 0, "MB session in"=w394) -> ("error out"=w389:errorcluster, "Coils"=w374:bool[], "MB session out"=w390:refnum<class "MB_Master.lvclass">)  [unwired: 5 in]
            n178 = global write "采配水全局变量.vi" "AD"(w409) -> ()
            n179 = formula code="float AD0,AD1,AD2,AD3,AD4,AD5,AD6;\n\nAD0 = IN[0]*140/6553-75;\nAD1 = IN[1]/65.53-25;\nAD2 = (IN[2]/65.53-25)/100;\nAD3 = IN[3]*30/8191;\nAD4 = IN[4]*30/8191;\nAD5 = IN[5]*30/8191;"("IN"=w370) -> ("AD0"=w407:dbl, "AD1"=w406:dbl, "AD2"=w350:dbl, "AD3"=w405:dbl, "AD4"=w404:dbl, "AD5"=w403:dbl)
            "压力传感器" <- w350
            n180 = global write "采配水全局变量.vi" "输出状态"(w374) -> ()
            n181 = call <vilib>:"Read Coils.vi"("error in (no error)"=w389, "quantity"=u16 16 ("number of coils"), "starting address"=u16 1000, "MB session in"=w390) -> ("error out"=w385:errorcluster, "Coils"=w381:bool[], "MB session out"=w386:refnum<class "MB_Master.lvclass">)  [unwired: 5 in]
            n182 = Index Array(array=w374, index #20=29 ("索引")) -> (element #1=w349:bool, element #2=w365:bool, element #3=w364:bool, element #4=w363:bool, element #5=w362:bool, element #6=w361:bool, element #7=w360:bool, element #8=w356:bool, element #9=w355:bool, element #10=w354:bool, element #11=w353:bool, element #12=w352:bool, element #13=w351:bool, element #14=w348:bool, element #15=w347:bool, element #16=w346:bool, element #17=w345:bool, element #18=w344:bool, element #19=w343:bool, element #20=w319:bool, element #21=w312:bool)  [unwired: 20 in]
            n183 = Bundle(w407, w406, w350, w405, w404, w403) -> (w408:cluster{dbl, dbl, dbl, dbl, dbl, dbl})  [unwired: 1 in]
            n184 = global write "采配水全局变量.vi" "输入状态"(w381) -> ()
            n185 = local write "Y0"(w349) -> ()
            n186 = local write "Y1"(w365) -> ()
            n187 = local write "Y2"(w364) -> ()
            n188 = local write "Y3"(w363) -> ()
            n189 = local write "Y4"(w362) -> ()
            n190 = local write "Y5"(w361) -> ()
            n191 = local write "Y6"(w360) -> ()
            n192 = local write "Y7"(w356) -> ()
            n193 = local write "Y8"(w355) -> ()
            n194 = local write "Y9"(w354) -> ()
            n195 = local write "Y10"(w353) -> ()
            n196 = local write "Y11"(w352) -> ()
            n197 = local write "Y12"(w351) -> ()
            n198 = local write "Y13"(w348) -> ()
            n199 = local write "Y14"(w347) -> ()
            n200 = local write "Y15"(w346) -> ()
            n201 = local write "Y16"(w345) -> ()
            n202 = local write "Y17"(w344) -> ()
            n203 = local write "Y18"(w343) -> ()
            n204 = local write "Y29"(w319) -> ()
            n205 = local write "Y30"(w312) -> ()
            n206 = call <vilib>:"Read Coils.vi"("error in (no error)"=w385, "quantity"=u16 16 ("number of coils"), "starting address"=u16 2500, "MB session in"=w386) -> ("error out"=w308:errorcluster, "Coils"=w382:bool[], "MB session out"=w318:refnum<class "MB_Master.lvclass">)  [unwired: 5 in]
            n207 = global write "采配水全局变量.vi" "转换值"(w408) -> ()
            n208 = Index Array(array=w381) -> (element #1=→"X0":bool, element #2=→"X1":bool, element #3=→"X2":bool, element #4=→"X3":bool, element #5=→"X4":bool, element #6=→"X5":bool, element #7=→"X6":bool, element #8=→"X7":bool, element #9=→"X8":bool, element #10=→"X9":bool, element #11=→"X10":bool)  [unwired: 12 in, 1 out]
            n209 = global write "采配水全局变量.vi" "报警簇"(w382) -> ()
            n210 = call <vilib>:"Read Coils.vi"("error in (no error)"=w308, "quantity"=u16 2, "starting address"=u16 2800, "MB session in"=w318) -> ("error out"=w307:errorcluster, "Coils"=w314:bool[], "MB session out"=w317:refnum<class "MB_Master.lvclass">)  [unwired: 5 in]
            n211 = Index Array(array=w314) -> (element #1=w313:bool, element #2=w309:bool)  [unwired: 2 in]
            n212 = local write "三级过滤系统"(w309) -> ()
            n213 = global write "采配水全局变量.vi" "看门狗启用"(w313) -> ()
          }
          frame "读参数" {
            n214 = call <vilib>:"Read Holding Registers.vi"("error in (no error)"=w436, "quantity"=u16 25 ("number of holding registers"), "starting address"=u16 100, "MB session in"=w437) -> ("error out"=w431:errorcluster, "Registers"=w433:u16[], "MB session out"=w432:refnum<class "MB_Master.lvclass">)  [unwired: 5 in]
            n215 = Array To Cluster(array=w433) -> (cluster=w424:T18)
            n216 = global write "采配水全局变量.vi" "参数设置"(w424) -> ()
            n217 = Unbundle(w424) -> ("Registers[0]"=w423:u16, "Registers[1]"=→"R101":u16, "Registers[2]"=→"R102":u16, "Registers[3]"=→"R103":u16, "Registers[4]"=→"R104":u16, "Registers[5]"=→"R105":u16, "Registers[6]"=→"R106":u16, "Registers[7]"=→"R107":u16, "Registers[8]"=→"R108":u16, "Registers[9]"=→"R109":u16, "Registers[10]"=→"R110":u16, "Registers[11]"=→"R111":u16, "Registers[12]"=→"R112":u16, "Registers[13]"=w420:u16, "Registers[16]"=→"R116":u16, "Registers[17]"=→"R117":u16, "Registers[20]"=→"R120":u16, "Registers[21]"=→"R121":u16, "Registers[22]"=→"R122":u16, "Registers[24]"=→"R124":u16)  [unwired: 5 out]
            n218 = local write "R100"(w423) -> ()
            n219 = local write "R113"(w420) -> ()
          }
          frame "多个写入" {
            n220 = Unbundle By Name(w443) -> ("数据"=w442:variant)
            n221 = Variant To Data(type=T13 {"starting address"=0, "holding register values"=[]}, Variant=w442) -> (data=w440:T13)  [unwired: 1 in, 1 out]
            n222 = Unbundle By Name(w440) -> ("starting address"=w439:u16, "holding register values"=w438:u16[])
            n223 = call <vilib>:"Write Multiple Registers.vi"("error in (no error)"=w446, "values"=w438, "starting address"=w439, "MB session in"=w447) -> ("error out"=w445:errorcluster, "MB session out"=w444:refnum<class "MB_Master.lvclass">)  [unwired: 6 in]
          }
          frame "单个写入" {
            n224 = Unbundle By Name(w453) -> ("数据"=w452:variant)
            n225 = Variant To Data(type=T14 {"starting address"=0, "holding register value"=0}, Variant=w452) -> (data=w450:T14)  [unwired: 1 in, 1 out]
            n226 = Unbundle By Name(w450) -> ("starting address"=w449:u16, "holding register value"=w448:u16)
            n227 = call <vilib>:"Write Single Register.vi"("error in (no error)"=w456, "value"=w448, "address"=w449, "MB session in"=w457) -> ("error out"=w455:errorcluster, "MB session out"=w454:refnum<class "MB_Master.lvclass">)  [unwired: 6 in]
          }
          frame "线圈写入" {
            n228 = Unbundle By Name(w463) -> ("数据"=w462:variant)
            n229 = Variant To Data(type=T15 {"starting address"=0, "coil values"=[]}, Variant=w462) -> (data=w460:T15)  [unwired: 1 in, 1 out]
            n230 = Unbundle By Name(w460) -> ("starting address"=w459:u16, "coil values"=w458:bool[])
            n231 = call <vilib>:"Write Multiple Coils.vi"("error in (no error)"=w466, "values"=w458, "starting address"=w459, "MB session in"=w467) -> ("error out"=w465:errorcluster, "MB session out"=w464:refnum<class "MB_Master.lvclass">)  [unwired: 6 in]
          }
          frame "shutdown" {
            n232 = call <vilib>:"Write Single Register.vi"("error in (no error)"=w475, "value"=u16 0, "address"=u16 4047, "MB session in"=w479) -> ("error out"=w474:errorcluster, "MB session out"=w478:refnum<class "MB_Master.lvclass">)  [unwired: 6 in]
            n233 = call-dynamic "Close Session.vi"("error in (no error)"=w474, "MB session in"=w478) -> ("error out"=w480:errorcluster)  [unwired: 9 in]
            n234 = call <vilib>:"Clear Errors.vi"("error in (no error)"=w480) -> ("error out"=w470:errorcluster)  [unwired: 5 in, 1 out]
            n235 = call "文件对话框"("start path"=path "D:/SRC", "pattern (all files)"="*.pdw", "pattern label"="PLC") -> ("selected path"=w473:path, "cancelled"=w471:bool)  [unwired: 9 in, 2 out]
            n236 = case shown="假" w471 {
              tunnel: w473 -> [w486 _]
              tunnel: w470 -> [_ _]
              frame False {
                n237 = Path To String(path=w486) -> (string=w483:string)
                n238 = Format Into String(format string="  - \"%s\"" ("格式字符串"), initial string="\"C:\\Program Files\\Fatek\\WinProladder\\WProlad.exe\"" ("command line"), w483) -> (resulting string=w484:string)  [unwired: 1 in, 1 out]
                n239 = call <vilib>:"System Exec.vi"("command line"=w484) -> ("error out"=w487:errorcluster)  [unwired: 7 in, 3 out]
                n240 = case shown="错误" w487 {
                  tunnel: w483 -> [_ w490]
                  frame No Error {
                  }
                  frame Error {
                    n241 = Format Into String(format string="  - \"%s\"" ("格式字符串"), initial string="\"C:\\Program Files (x86)\\Fatek\\WinProladder\\WProlad.exe\"" ("command line"), w490) -> (resulting string=w488:string)  [unwired: 1 in, 1 out]
                    n242 = call <vilib>:"System Exec.vi"("command line"=w488) -> ()  [unwired: 7 in, 4 out]
                  }
                }
              }
              frame True {
              }
            }
          }
        }
      }
      frame Error {
        n243 = Unbundle By Name(w496) -> ("code"=w498:i32)
        n244 = case shown="-1073807343" w498 {
          tunnel: w497 -> [w500 w504]
          tunnel: w496 -> [w499 w506]
          tunnel: [w499 w505] -> w494
          tunnel: [w500 w504] -> w495
          tunnel: w492 -> [_ w503]
          frame Default {
          }
          frame -1073807343 {
            n245 = Flush Queue(queue=w503) -> (queue out=w502:refnum<queue>)  [unwired: 1 in, 2 out]
            n246 = call-dynamic "Close Session.vi"("error in (no error)"=w506, "MB session in"=w504) -> ("error out"=w505:errorcluster)  [unwired: 9 in]
            n247 = disable-structure shown="禁用" {
              disable-tunnel: w502 -> [w507 _]
              frame Disabled {
                n248 = Enqueue Element At Opposite End(queue=w507, element=cluster{"命令":string, "数据":variant} {"命令"="init", "数据"=variant} ("元素")) -> ()  [unwired: 2 in, 3 out]
              }
              frame Enabled {
              }
            }
            n249 = Wait (ms)(milliseconds to wait=u32 2000 ("等待时间（毫秒）")) -> ()  [unwired: 1 out]
          }
        }
        n250 = call <vilib>:"Clear Errors.vi"("error in (no error)"=w494) -> ("error out"=w493:errorcluster)  [unwired: 5 in, 1 out]
      }
    }
    n251 = Unbundle By Name(w272) -> ("status"=→"通讯故障":bool)
  }
  n252 = property on="多列列表框" class="MCListbox (严格)"("ItemNames"=string[][] [["待机"], ["初始化"], ["水样润洗"], ["一级水样池进样"], ["二级水样池进样"], ["沉淀/三级水样池进样"], ["配水"], ["反冲洗"], ["一级采样池储水"], ["结束"]] ("项名")) -> ()  [unwired: 2 in, 2 out]
  n253 = call-dynamic "Close Session.vi"("error in (no error)"=w6, "MB session in"=w5) -> ()  [unwired: 9 in, 1 out]
